vi "Compile Knock Cylinder 1.0 Data.vi"(8 "error in (no error)":errorcluster, 11 "Device Item Ref in":T3 format="%.0x") -> (0 "error out":errorcluster, 2 "Knock Cylinders":T1[](array[typedef]), 3 "Device Item Ref out":T3 format="%.0x")   [LabVIEW 2013, in "Engine Simulation Toolkit System Explorer.lvlib"]
uses:
  Engine Simulation Toolkit System Explorer.lvlib
  <vilib>/NI Veristand/Custom Device API/Custom Device Item Ref.ctl
  Shared/1.0 Knock Cylinder Engine Data.ctl
  Shared/1.0 Knock Cylinder FIFO Idxs.ctl
  Shared/Constants and GUIDs.vi
  <vilib>/NI Veristand/Custom Device Tools/Custom Device Utility Library/NI VeriStand - Search for All Items by GUID.vi
  Shared/Properties.vi
  <vilib>/NI Veristand/Custom Device API/Get Item Property (Double).vi
  <vilib>/NI Veristand/Custom Device API/Get Item Property (String).vi
  Shared/Engine Simulation Toolkit Shared.lvlib
  <vilib>/NI Veristand/Custom Device Tools/Custom Device Utility Library/Custom Device Utility Library.lvlib
  <vilib>/NI Veristand/Custom Device API/Custom Device API.lvlib
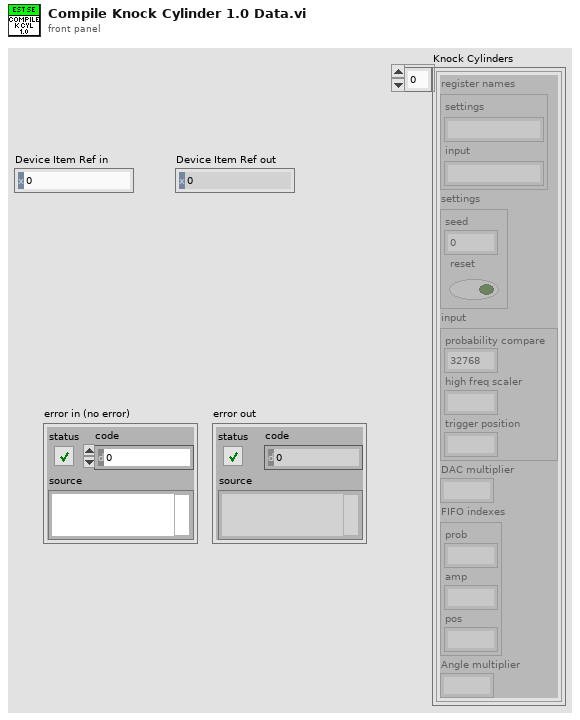
[diagram p1: front panel]
types:
  T1 = typedef "Engine Simulation Toolkit Shared.lvlib/1.0 Knock Cylinder Engine Data.ctl" = cluster{"register names":cluster{"settings":string, "input":string}, "settings":cluster{"seed":u16, "reset":bool}, "input":cluster{"probability compare":u16, "high freq scaler":fxp<+,10,0>, "trigger position":u16}, "DAC multiplier":dbl, "FIFO indexes":T2, "Angle multiplier":dbl}
  T2 = typedef "Engine Simulation Toolkit Shared.lvlib/1.0 Knock Cylinder FIFO Idxs.ctl" = cluster{"prob":i32, "amp":i32, "pos":i32}
  T3 = typedef "Custom Device API.lvlib/Custom Device Item Ref.ctl" = u64
  T4 = typedef "Engine Simulation Toolkit Shared.lvlib/Channel.ctl" = cluster{"Name":string, "Units":string, "Default":dbl, "Description":string}
  T5 = typedef "Engine Simulation Toolkit System Explorer.lvlib/Knock Cylinder.ctl" = cluster{"Name":string, "Bitfile name":string, "Probability":dbl, "Amplitude":dbl, "Angle":dbl}
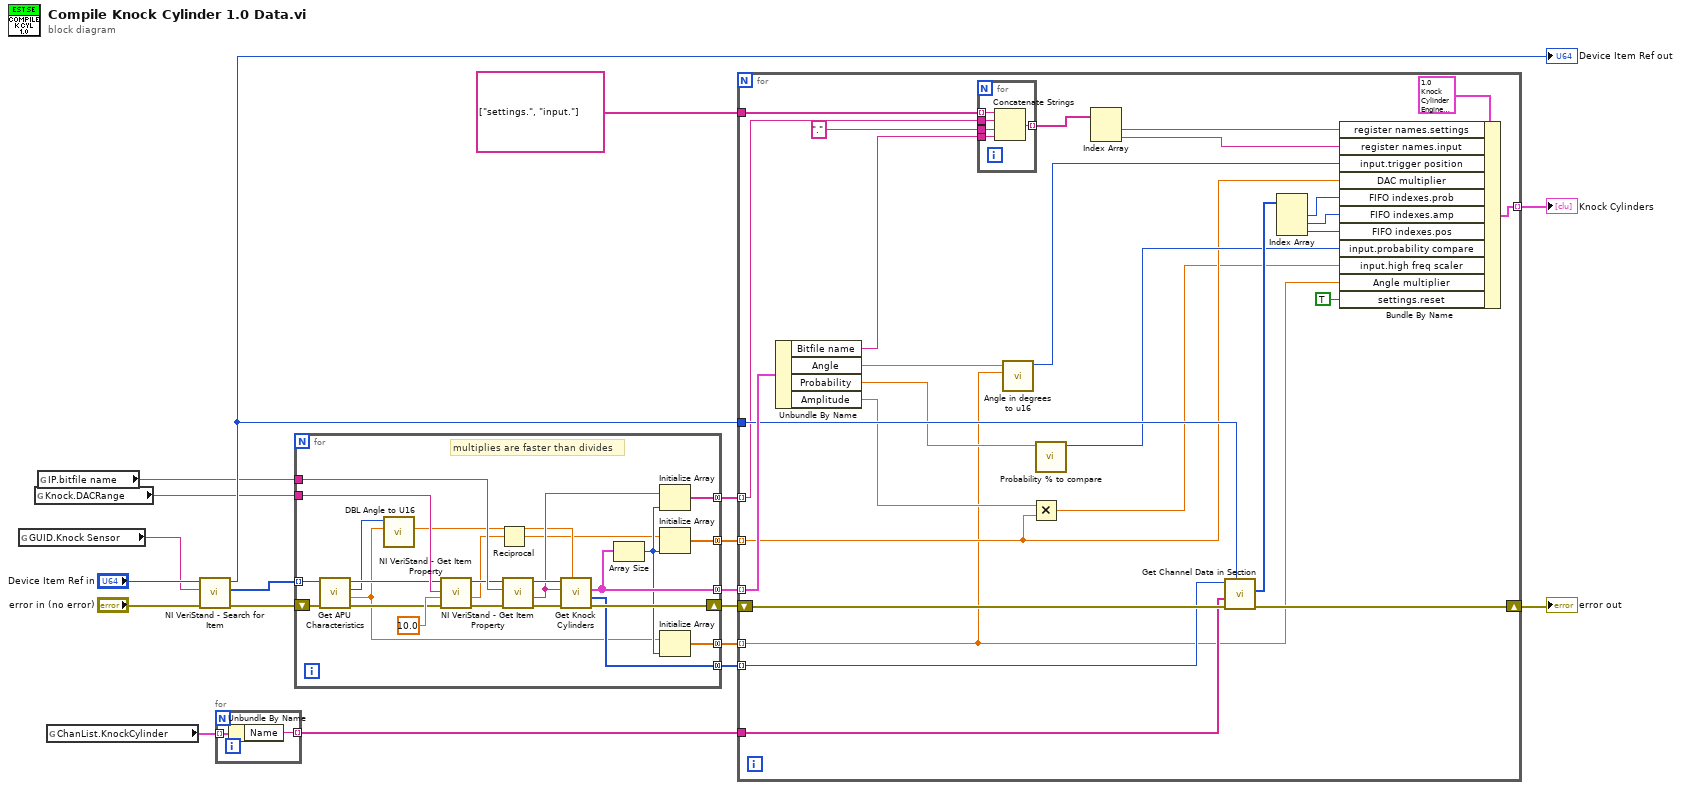
[diagram p0: block diagram]
diagram:
  n1 = global read "Constants and GUIDs.vi" "GUID.Knock Sensor"() -> (w10:string)
  n2 = global read "Properties.vi" "Knock.DACRange"() -> (w7:string)
  n3 = global read "Properties.vi" "IP.bitfile name"() -> (w6:string)
  n4 = global read "Constants and GUIDs.vi" "ChanList.KnockCylinder"() -> (w12:T4[])
  n5 = call-poly <vilib>:"NI VeriStand - Search for Item.vi"("error in"="error in (no error)", "Item GUID"=w10, "Section Ref in"="Device Item Ref in") -> ("error out"=w17:errorcluster, "Item Refs"=w8:T3[], "Section Ref out"=w13:T3)  [unwired: 5 in, 1 out]
  "Device Item Ref out" <- w13
  n6 = for {
    tunnel: w12 -> [w21] mode=indexing
    tunnel: [w20] -> w11 mode=indexing
    n7 = Unbundle By Name(w21) -> ("Name"=w20:string)
  }
  n8 = for {
    tunnel: w8 -> [w29] mode=indexing
    shift-right: [w40] -> w9
    shift-left: w17 -> [w45]
    tunnel: w7 -> [w42]
    tunnel: w6 -> [w41]
    tunnel: [w38] -> w5 mode=concatenating
    tunnel: [w33] -> w4 mode=concatenating
    tunnel: [w37] -> w3 mode=concatenating
    tunnel: [w36] -> w2 mode=concatenating
    tunnel: [w23] -> w1 mode=concatenating
    # "multiplies are faster than divides"
    n9 = call "Get APU Characteristics.vi"("error in (no error)"=w45, "Item Ref in"=w29) -> ("error out"=w30:errorcluster, "angle to u16 scale factor"=w24:dbl, "total angle span (degrees)"=w27:u16, "Item Ref out"=w28:T3)  [unwired: 3 in, 3 out]
    n10 = call "DBL Angle to U16.vi"("angle to u16 scale factor"=w24, "Desired angle (degrees)"=w27) -> ("Actual angle (degrees)"=w26:dbl)  [unwired: 8 in, 1 out]
    n11 = call-poly <vilib>:"NI VeriStand - Get Item Property.vi"("error in (no error)"=w30, "Default Value"=10.0, "Property Name"=w42, "Item Ref in"=w28) -> ("error out"=w44:errorcluster, "Value"=w31:dbl, "Item Ref out"=w35:T3)  [unwired: 4 in, 1 out]
    n12 = Reciprocal(x=w31) -> (1/x=w22:dbl)
    n13 = call-poly <vilib>:"NI VeriStand - Get Item Property.vi"("error in (no error)"=w44, "Property Name"=w41, "Item Ref in"=w35) -> ("error out"=w43:errorcluster, "Value"=w34:string, "Item Ref out"=w39:T3)  [unwired: 5 in, 1 out]
    n14 = call "Get Knock Cylinders.vi"("Max angle"=w26, "error in (no error)"=w43, "Knock Sensor"=w34, "Item Ref in"=w39) -> ("error out"=w40:errorcluster, "cylinder item refs"=w33:T3[], "cylinders"=w38:T5[])  [unwired: 3 in, 2 out]
    n15 = Array Size(array=w38) -> (size(s)=w25:i32)
    n16 = Initialize Array(w34, w25) -> (w36:string[])
    n17 = Initialize Array(w22, w25) -> (w37:dbl[])
    n18 = Initialize Array(w24, w25) -> (w23:dbl[])
  }
  n19 = for {
    shift-right: [w62] -> w15
    shift-left: w9 -> [w66]
    tunnel: string[] ["settings.", "input."] -> [w73]
    tunnel: w11 -> [w63]
    tunnel: [w71] -> w14 mode=indexing
    tunnel: w13 -> [w64]
    tunnel: w5 -> [w70] mode=indexing
    tunnel: w4 -> [w65] mode=indexing
    tunnel: w3 -> [w50] mode=indexing
    tunnel: w2 -> [w59] mode=indexing
    tunnel: w1 -> [w47] mode=indexing
    n20 = Unbundle By Name(w70) -> ("Bitfile name"=w69:string, "Angle"=w57:dbl, "Probability"=w53:dbl, "Amplitude"=w51:dbl)
    n21 = for {
      tunnel: w73 -> [w78] mode=indexing
      tunnel: [w74] -> w68 mode=indexing
      tunnel: w69 -> [w77]
      tunnel: w59 -> [w76]
      tunnel: "." -> [w75]
      n22 = Concatenate Strings(w78, w76, w75, w77) -> (w74:string)
    }
    n23 = call "Angle in degrees to u16.vi"("angle to u16 scale factor"=w47, "Angle (deg)"=w57) -> ("u16 angle"=w56:u16)  [unwired: 8 in, 1 out]
    n24 = Multiply(x=w51, y=w50) -> (x*y=w49:dbl)
    n25 = call "Probability % to compare.vi"("probability %"=w53) -> ("probability compare"=w52:u16)  [unwired: 10 in]
    n26 = Index Array(array=w68) -> (element #1=w67:string, element #2=w58:string)  [unwired: 2 in]
    n27 = call "Get Channel Data in Section.vi"("Custom device ref"=w64, "error in (no error)"=w66, "Channels"=w63, "Item Ref in"=w65) -> ("error out"=w62:errorcluster, "FIFO indexes"=w61:i32[])  [unwired: 3 in, 3 out]
    n28 = Index Array(array=w61) -> (element #1=w55:i32, element #2=w54:i32, element #3=w48:i32)  [unwired: 3 in]
    n29 = Bundle By Name(cluster=T1 {"register names"={"settings"="", "input"=""}, "settings"={"seed"=0, "reset"=FALSE}, "input"={"probability compare"=32768, "high freq scaler"=0.0, "trigger position"=0}, "DAC multiplier"=0.0, "FIFO indexes"={"prob"=0, "amp"=0, "pos"=0}, "Angle multiplier"=0.0} ("1.0.0 Knock Cylinder"), "register names.settings"=w67, "register names.input"=w58, "input.trigger position"=w56, "DAC multiplier"=w50, "FIFO indexes.prob"=w55, "FIFO indexes.amp"=w54, "FIFO indexes.pos"=w48, "input.probability compare"=w52, "input.high freq scaler"=w49, "Angle multiplier"=w47, "settings.reset"=TRUE) -> (w71:T1)
  }
  "error out" <- w15
  "Knock Cylinders" <- w14
